vi "N4_X01_write_mode.vi"(4 "Driver Name":T10, 6 "Error Code":T11, 7 "Command":T8, 8 "error in":T9, 11 "DriverConnect in":T1={"InterfaceType"=enum."VISA", "OpenedSession"="", "InterfaceSettings"={"Interface"=enum."RS232", "EOS 4 read"=enum."LF (\\n)", "EOS 4 write"=enum."LF (\\n)", "TMO, ms"=10000, "Sett"=variant(cluster{"Baud Rate":u32, "Data Bits":u16, "Parity":u16, "Stop Bits":u16, "Flow Control":u16, "Eho":bool} {"Baud Rate"=75, "Data Bits"=0, "Parity"=0, "Stop Bits"=0, "Flow Control"=0, "Eho"=FALSE})}}) -> (0 "error out":T9, 3 "DriverConnect out":T1={"InterfaceType"=enum."VISA", "OpenedSession"="", "InterfaceSettings"={"Interface"=enum."RS232", "EOS 4 read"=enum."LF (\\n)", "EOS 4 write"=enum."LF (\\n)", "TMO, ms"=10000, "Sett"=variant(cluster{"Baud Rate":u32, "Data Bits":u16, "Parity":u16, "Stop Bits":u16, "Flow Control":u16, "Eho":bool} {"Baud Rate"=75, "Data Bits"=0, "Parity"=0, "Stop Bits"=0, "Flow Control"=0, "Eho"=FALSE})}}, 5 "ModeWasChacged":T6)   [LabVIEW 2018]
uses:
  MOKO_LabViewLibrary/MokoLowLevel/MokoLowLovelControl/MLLC_ErrorCode.ctl
  MOKO_LabViewLibrary/MokoLowLevel/MokoLowLovelControl/MLLC_DriverName.ctl
  MOKO_LabViewLibrary/MokoLowLevel/MokoLowLovelControl/MLLC_Error.ctl
  MOKO_LabViewLibrary/MokoLowLevel/MokoLowLovelControl/MLLC_Command.ctl
  MOKO_LabViewLibrary/MokoLowLevel/MokoLowLovelControl/MLLC_Delay.ctl
  MOKO_LabViewLibrary/MokoLowLevel/MokoLowLovelControl/MLLC_Boolean.ctl
  MOKO_LabViewLibrary/MokoLowLevel/MokoLowLovelControl/MLLC_ConnectCluster.ctl
  MOKO_LabViewLibrary/MokoLowLevel/MokoLowLovelControl/MLLC_InterfaceType.ctl
  MOKO_LabViewLibrary/MokoLowLevel/MokoLowLovelControl/MLLC_OpenedSession.ctl
  MOKO_LabViewLibrary/MokoLowLevel/MokoLowLovelControl/MLLC_InterfaceSettings.ctl
  MOKO_LabViewLibrary/MokoLowLevel/MokoLowLovelControl/MLLC_InterfaceKind.ctl
panel:
  in  "Delay Time (s)":T7=3.0
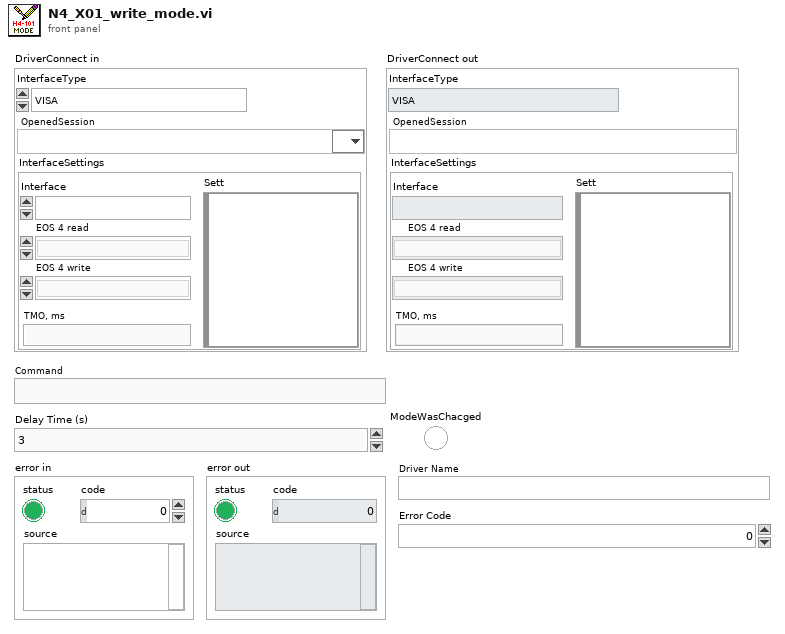
[diagram p1: front panel]
types:
  T1 = typedef "MLLC_ConnectCluster.ctl" = cluster{"InterfaceType":T2, "OpenedSession":T3, "InterfaceSettings":T4}
  T2 = typedef "MLLC_InterfaceType.ctl" = enum16{"VISA", "Prologix USB-GPIB"}
  T3 = typedef "MLLC_OpenedSession.ctl" = refnum<visa-resource-name>
  T4 = typedef "MLLC_InterfaceSettings.ctl" = cluster{"Interface":T5, "EOS 4 read":enum16{"Default (=EOS 4 write)", "CR (\\r)", "LF (\\n)", "None"}, "EOS 4 write":enum16{"CR+LF (\\r\\n)", "CR (\\r)", "LF (\\n)", "None"}, "TMO, ms":i32, "Sett":variant}
  T5 = typedef "MLLC_InterfaceKind.ctl" = enum16{"RS232", "GPIB", "USB", "Ethernet", "another"}
  T6 = typedef "MLLC_Boolean.ctl" = bool
  T7 = typedef "MLLC_Delay.ctl" = dbl
  T8 = typedef "MLLC_Command.ctl" = string
  T9 = typedef "MLLC_Error.ctl" = errorcluster
  T10 = typedef "MLLC_DriverName.ctl" = string
  T11 = typedef "MLLC_ErrorCode.ctl" = u32
  T12 = typedef "MLLC_Response.ctl" = string
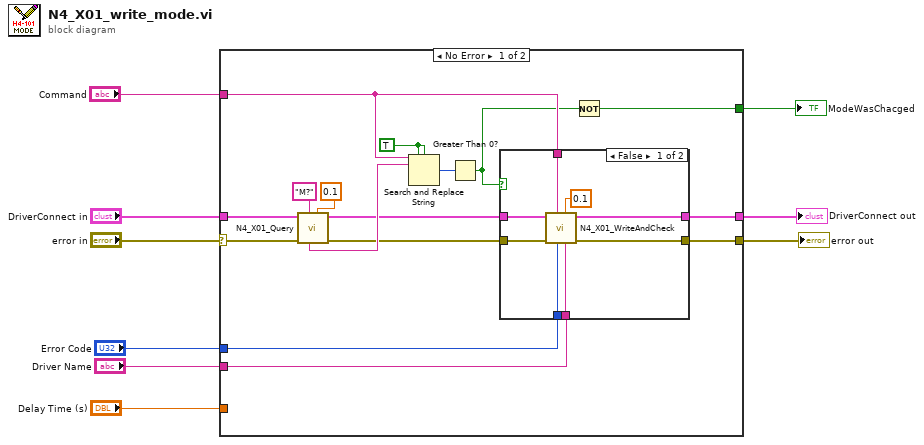
[diagram p0: block diagram]
diagram:
  n1 = case shown="No Error" "error in" {
    selector: "error in" -> [w19 w37]
    tunnel: [w22 w37] -> w9
    tunnel: [w23 w36] -> w1
    tunnel: "Error Code" -> [w25 _]
    tunnel: "Driver Name" -> [w24 _]
    tunnel: "DriverConnect in" -> [w20 w36]
    tunnel: "Command" -> [w18 _]
    tunnel: "Delay Time (s)" -> [_ _]
    tunnel: [w15 _] -> w3
    frame No Error {
      w17 = TRUE ("replace all? (F)")
      n2 = call "N4_X01_Query.vi"("Delay Befor (s)"=0.1 ("Command Time (s)"), "Command"="M?" ("Error Query"), "error in"=w19, "DriverConnect in"=w20) -> ("error out"=w11:T9, "DriverConnect out"=w12:T1, "Response"=w13:T12)  [unwired: 5 in]
      n3 = Search and Replace String(replace all?=w17, case sensitive?=w17, input string=w18, search string=w13) -> (number of replacements=w16:i32)  [unwired: 4 in, 3 out]
      n4 = Greater Than 0?(x=w16) -> (x > 0?=w14:bool)
      n5 = case shown="False" w14 {
        tunnel: w25 -> [w33 _]
        tunnel: w24 -> [w32 _]
        tunnel: [w31 w35] -> w23
        tunnel: [w27 w34] -> w22
        tunnel: w18 -> [w30 _]
        tunnel: w12 -> [w29 w35]
        tunnel: w11 -> [w28 w34]
        frame False {
          n6 = call "N4_X01_WriteAndCheck.vi"("Driver Name"=w32, "Command Time (s)"=0.1, "Error Code"=w33, "Command"=w30, "error in"=w28, "DriverConnect in"=w29) -> ("error out"=w27:T9, "DriverConnect out"=w31:T1)  [unwired: 4 in]
        }
        frame True {
        }
      }
      n7 = Not(x=w14) -> (.not. x?=w15:bool)
    }
    frame Error {
    }
  }
  "error out" <- w9
  "ModeWasChacged" <- w3
  "DriverConnect out" <- w1
